vi "Node - Create Channels.vi"(8 "error in (no error)":errorcluster, 10 "Item Ref In":T1=18446744073709551615 format="%.0x") -> (0 "error out":errorcluster)   [LabVIEW 2016]
uses:
  <vilib>/NI Veristand/Custom Device API/Custom Device API.lvlib
  <vilib>/NI Veristand/Custom Device API/Custom Device Item Ref.ctl
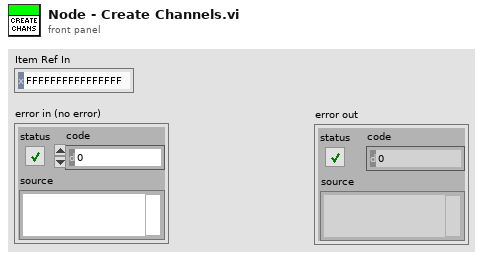
[diagram p1: front panel]
types:
  T1 = typedef "Custom Device API.lvlib/Custom Device Item Ref.ctl" = u64
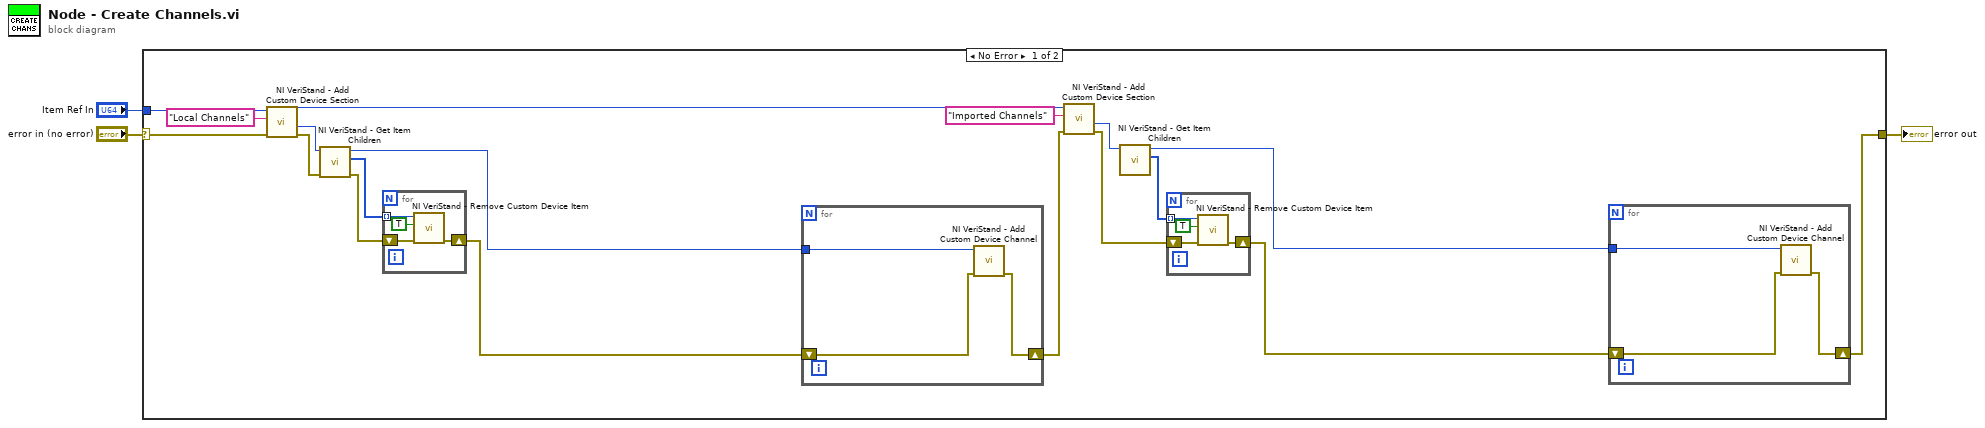
[diagram p0: block diagram]
diagram:
  n1 = case shown="No Error" "error in (no error)" {
    selector: "error in (no error)" -> [w16 w36]
    tunnel: "Item Ref In" -> [w21 _]
    tunnel: [w15 w36] -> w1
    frame No Error {
      n2 = call <vilib>:"NI VeriStand - Add Custom Device Section.vi"("error in (no error)"=w16, "Section Name"="Local Channels", "Parent Ref in"=w21) -> ("error out"=w11:errorcluster, "Section Ptr"=w14:T1, "Parent Ref out"=w19:T1)  [unwired: 5 in, 1 out]
      n3 = call <vilib>:"NI VeriStand - Get Item Children.vi"("error in (no error)"=w11, "Item Ref in"=w14) -> ("error out"=w10:errorcluster, "Child Refs"=w12:T1[], "Item Ref out"=w13:T1)  [unwired: 6 in, 1 out]
      n4 = for {
        tunnel: w12 -> [w28] mode=indexing
        shift-right: [w26] -> w9
        shift-left: w10 -> [w27]
        n5 = call <vilib>:"NI VeriStand - Remove Custom Device Item.vi"("error in (no error)"=w27, "Force Delete (F)"=TRUE, "Item Ref in"=w28) -> ("error out"=w26:errorcluster)  [unwired: 7 in, 1 out]
      }
      n6 = for {
        shift-right: [w33] -> w20
        shift-left: w9 -> [w34]
        tunnel: w13 -> [w35]
        n7 = call <vilib>:"NI VeriStand - Add Custom Device Channel.vi"("error in (no error)"=w34, "Parent Ref in"=w35) -> ("error out"=w33:errorcluster)  [unwired: 6 in, 3 out]
      }
      n8 = call <vilib>:"NI VeriStand - Add Custom Device Section.vi"("error in (no error)"=w20, "Section Name"="Imported Channels", "Parent Ref in"=w19) -> ("error out"=w8:errorcluster, "Section Ptr"=w6:T1)  [unwired: 5 in, 2 out]
      n9 = call <vilib>:"NI VeriStand - Get Item Children.vi"("Item Ref in"=w6) -> ("Child Refs"=w5:T1[], "Item Ref out"=w4:T1)  [unwired: 7 in, 2 out]
      n10 = for {
        tunnel: w5 -> [w24] mode=indexing
        shift-right: [w22] -> w7
        shift-left: w8 -> [w23]
        n11 = call <vilib>:"NI VeriStand - Remove Custom Device Item.vi"("error in (no error)"=w23, "Force Delete (F)"=TRUE, "Item Ref in"=w24) -> ("error out"=w22:errorcluster)  [unwired: 7 in, 1 out]
      }
      n12 = for {
        shift-right: [w30] -> w15
        shift-left: w7 -> [w31]
        tunnel: w4 -> [w32]
        n13 = call <vilib>:"NI VeriStand - Add Custom Device Channel.vi"("error in (no error)"=w31, "Parent Ref in"=w32) -> ("error out"=w30:errorcluster)  [unwired: 6 in, 3 out]
      }
    }
    frame Error {
    }
  }
  "error out" <- w1
